vi "Get uptime.vi"(8 "error in (no error)":errorcluster, 11 "AlphaStep One in":refnum<class "AlphaStep One.lvclass">) -> (0 "error out":errorcluster, 2 "Uptime (sec)":dbl, 3 "AlphaStep One out":refnum<class "AlphaStep One.lvclass">)   [LabVIEW 2019, in "AlphaStep One.lvclass"]
uses:
  AlphaStep One.lvclass
  AlphaStep One.lvclass/AlphaStep One.ctl
  Serial Device/Serial Device.lvclass
panel:
  out "RX Data":string
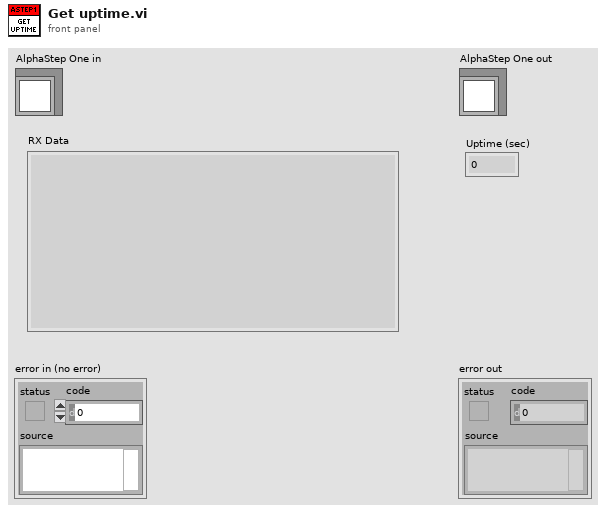
[diagram p1: front panel]
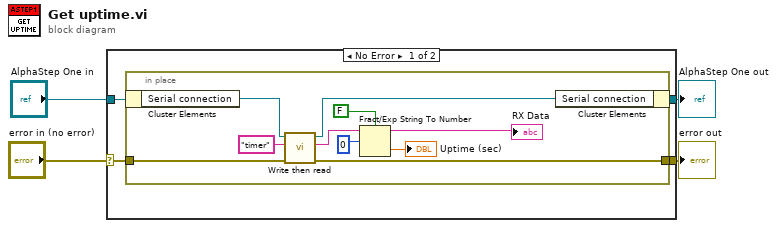
[diagram p0: block diagram]
diagram:
  n1 = case shown="No Error" "error in (no error)" {
    selector: "error in (no error)" -> [w6 w19]
    tunnel: [w5 w19] -> w3
    tunnel: "AlphaStep One in" -> [w8 w18]
    tunnel: [w7 w18] -> w1
    frame No Error {
      n2 = in-place {
        in-place-border: w6 -> [w15]
        in-place-border: [w14] -> w5
        n3 = in-place-cluster #1(w8) -> ("Serial connection"=w17:refnum<class "Serial Device.lvclass">)
        n4 = call "Write then read.vi"("error in (no error)"=w15, "TX Data"="timer", "Serial Device in"=w17) -> ("error out"=w14:errorcluster, "RX Data"=w11:string, "Serial Device out"=w16:refnum<class "Serial Device.lvclass">)  [unwired: 6 in]
        "RX Data" <- w11
        n5 = Fract/Exp String To Number(use system decimal point (T)=FALSE, string=w11, offset=0) -> (number=→"Uptime (sec)":dbl)  [unwired: 1 in, 1 out]
        n6 = in-place-cluster #1("Serial connection"=w16) -> (w7:refnum<class "AlphaStep One.lvclass">)
      }
    }
    frame Error {
    }
  }
  "error out" <- w3
  "AlphaStep One out" <- w1
